vi "test6-AsteriskWildcardStatusRegistration.vi"(8 "error in (no error)":errorcluster, 11 "TestCase in":refnum<class "testcase-CSMBroadcast.lvclass">) -> (0 "error out":errorcluster, 3 "TestCase out":refnum<class "testcase-CSMBroadcast.lvclass">)   [LabVIEW 2017, in "testcase-CSMBroadcast.lvclass"]
uses:
  testcase-CSMBroadcast.lvclass
  0c20cacf-7d77-4f8e-aec5-f22e7d09936d.vi
  26de337d-8090-412f-9da5-e117a55d4726.vi
  de10340a-d592-45ad-b055-7fa7b377c551.vi
  e3eae2f8-d8ce-4adb-8167-9a417250fce1.vi
  a4d00e00-a9ed-4631-bf53-269bf71f16fc.vi
  src/user.lib/_NEVSTOP/Communicable State Machine(CSM)/AdvanceAPI/CSM - Revert Arguments-Safe String.vi
  src/user.lib/_NEVSTOP/Communicable State Machine(CSM)/AdvanceAPI/CSM - Make String Arguments Safe.vi
  src/user.lib/_NEVSTOP/Communicable State Machine(CSM)/AdvanceAPI/CSM - Break Down Multiple States String.vi
  src/user.lib/_NEVSTOP/Communicable State Machine(CSM)/AdvanceAPI/CSM - Compact Multiple States.vi
  src/user.lib/_NEVSTOP/Communicable State Machine(CSM)/AdvanceAPI/CSM - Keywords.vi
  src/user.lib/_NEVSTOP/Communicable State Machine(CSM)/_Shared/Trim Single-line Text.vi
  src/user.lib/_NEVSTOP/Communicable State Machine(CSM)/AdvanceAPI/CSM - Set Module Attribute.vi
  src/user.lib/_NEVSTOP/Communicable State Machine(CSM)/AdvanceAPI/CSM - Get Module Attribute.vi
  <vilib>/addons/_JKI Toolkits/VI Tester/TestCase.llb/TestCase.lvclass
  src/user.lib/_NEVSTOP/Communicable State Machine(CSM)/Communicable State Machine.lvlib
  CSM/CSM-Testcase.lvlib
  C:/Program Files (x86)/National Instruments/LabVIEW 2017/vi.lib/addons/_JKI Toolkits/VI Tester/TestCase.llb/TestCase.lvclass
panel:
  out "Execution Times":i32
  out "State History":string
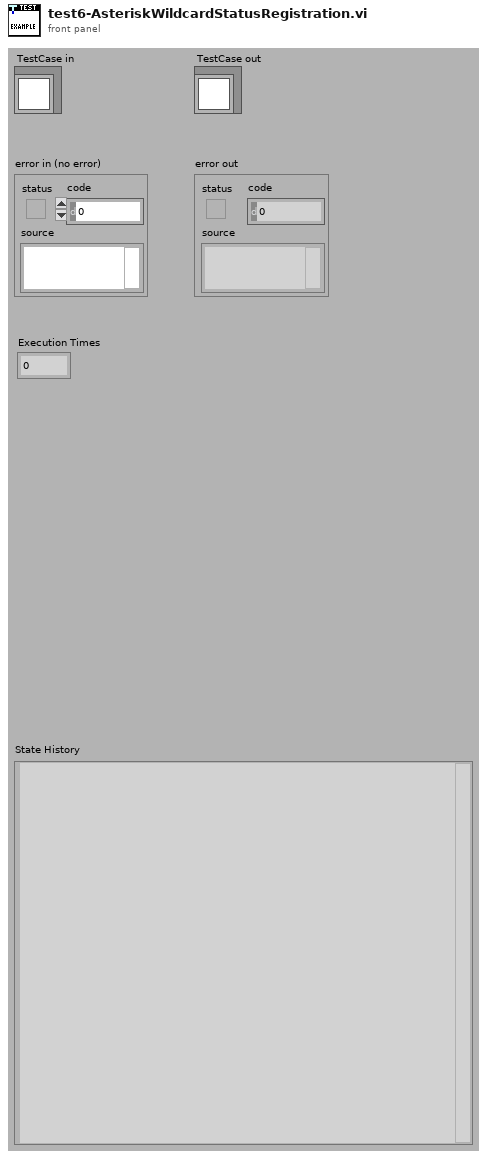
[diagram p1: front panel]
types:
  T1 = enum32{"Invalid", "Standard", "Closed", "Hidden", "Minimized", "Maximized"}
  T2 = enum32{"invalid app kind", "Development System", "Run Time System", "Student Edition", "Embedded LabVIEW", "Evaluation", "Custom"}
  T3 = typedef "Communicable State Machine.lvlib/_CSM_Response Source Message.ctl" = cluster{"‘State":string, "’Arguments":string, "’Error":errorcluster}
  T4 = cluster{"Current VI Reference":refnum<vi>, "Close Panel on Exit?":bool}
  T5 = cluster{"Core":cluster{"Current VI Reference":refnum<vi>, "Close Panel on Exit?":bool}, "Your Boolean data":bool, "Your string data":string, "TestData":i32}
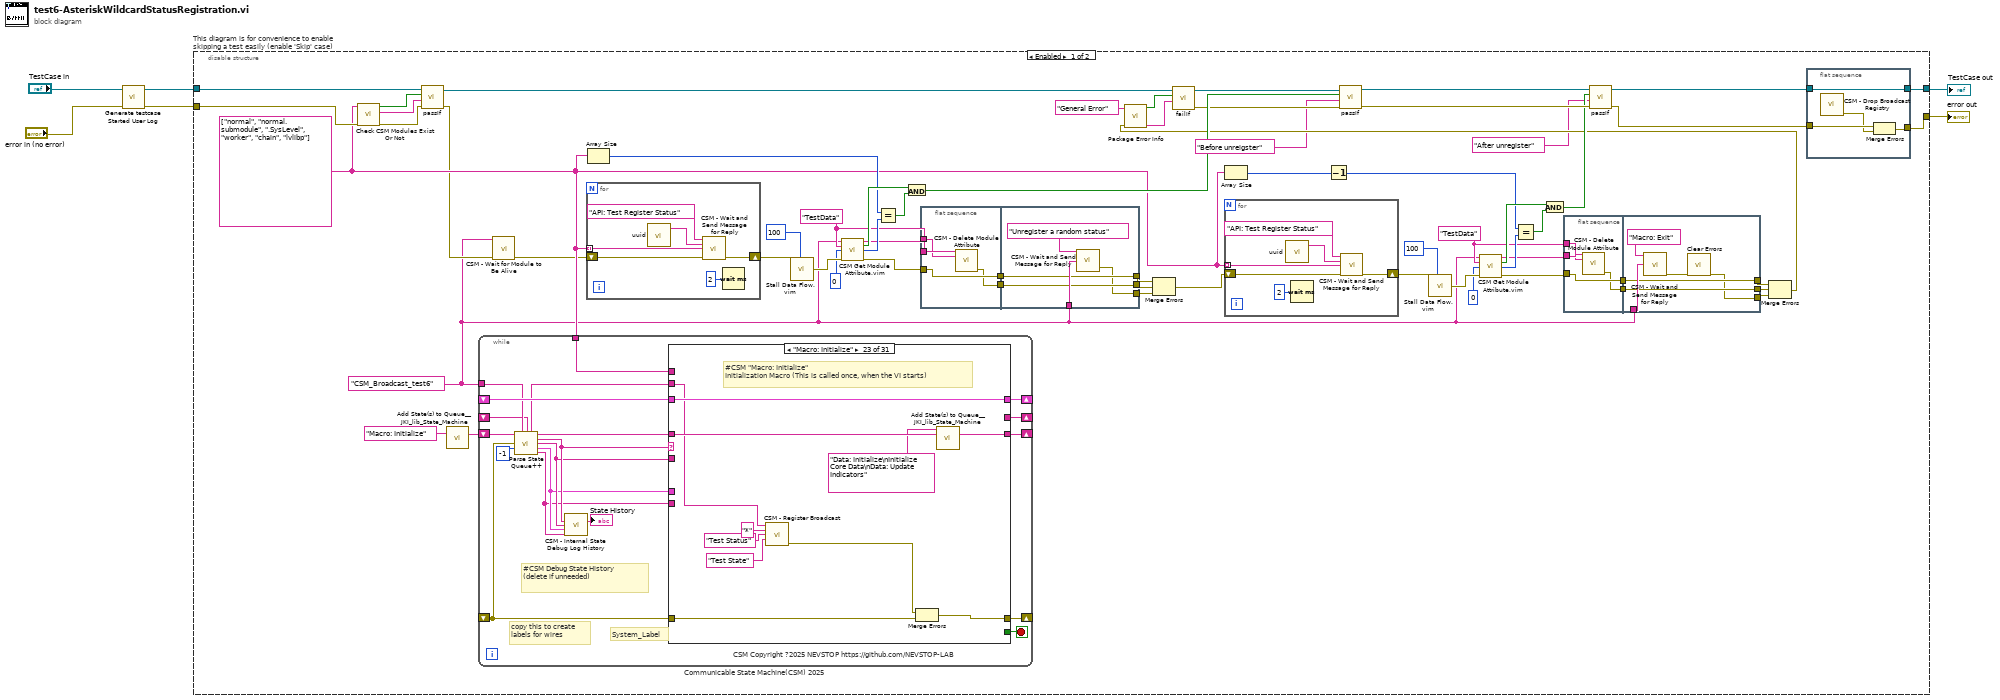
[diagram p0: block diagram]
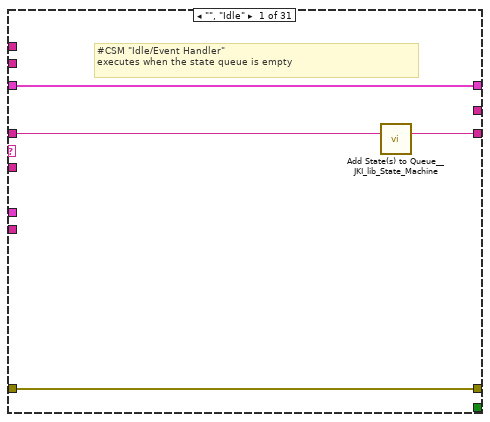
[diagram p2: hidden frame]
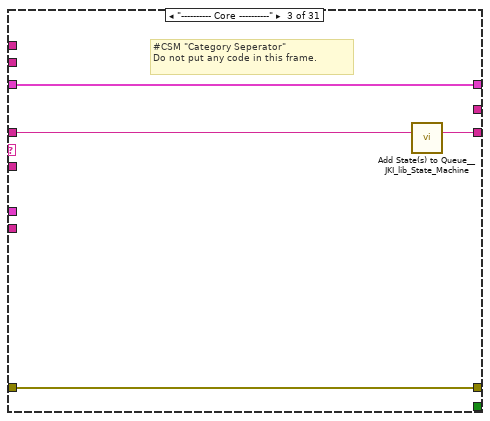
[diagram p4: hidden frame]
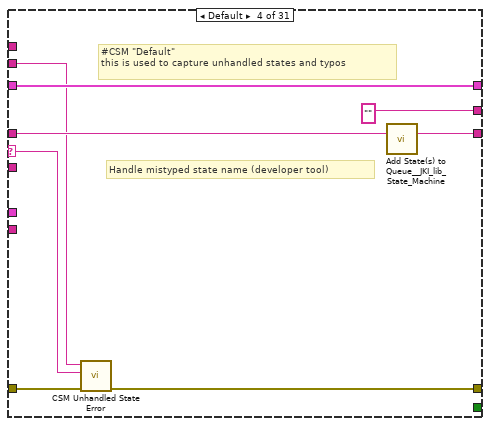
[diagram p5: hidden frame]
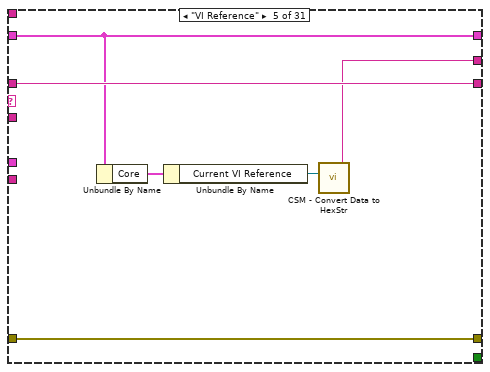
[diagram p6: hidden frame]
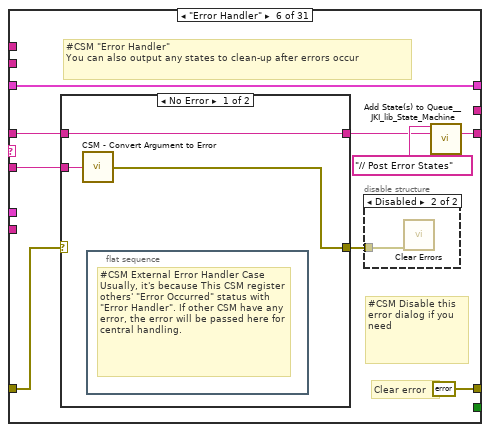
[diagram p7: hidden frame]
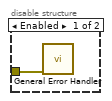
[diagram p8: hidden frame]
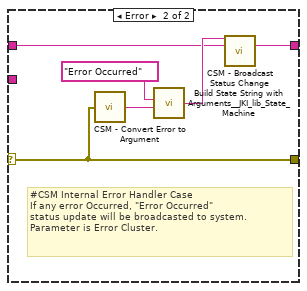
[diagram p9: hidden frame]
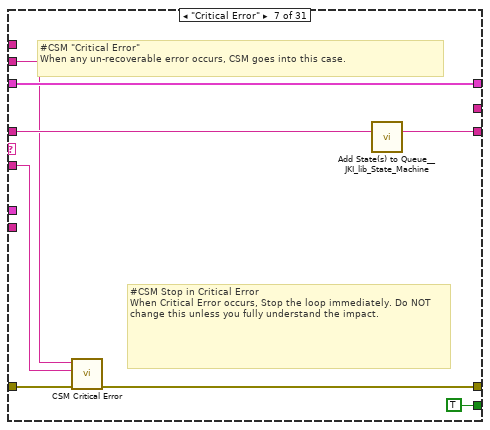
[diagram p10: hidden frame]
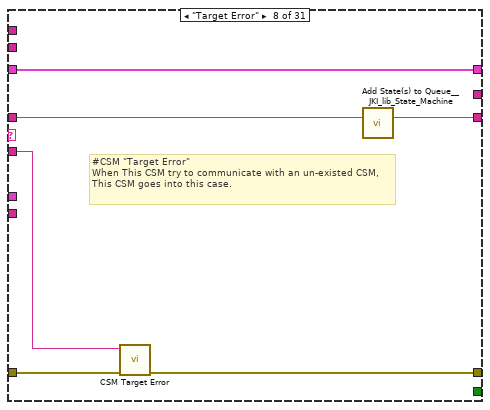
[diagram p11: hidden frame]
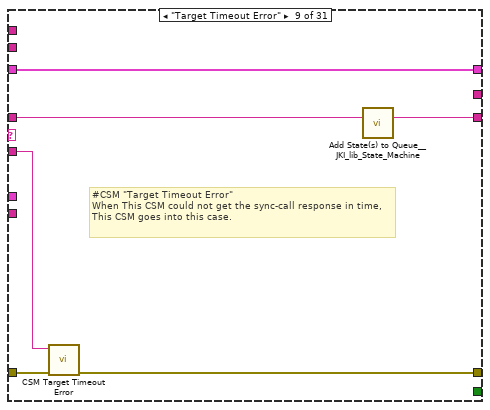
[diagram p12: hidden frame]
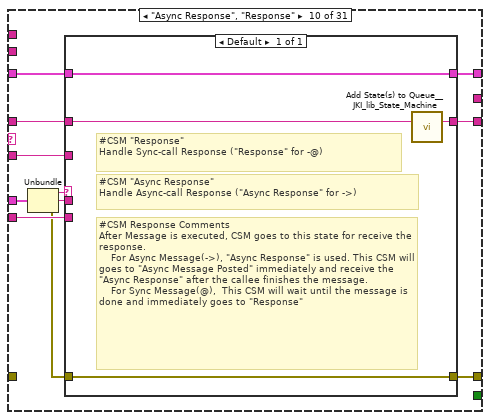
[diagram p13: hidden frame]
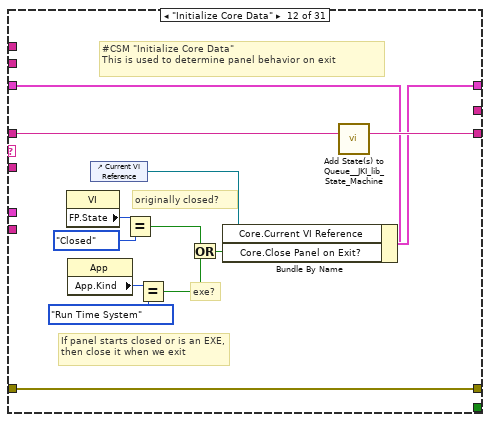
[diagram p15: hidden frame]
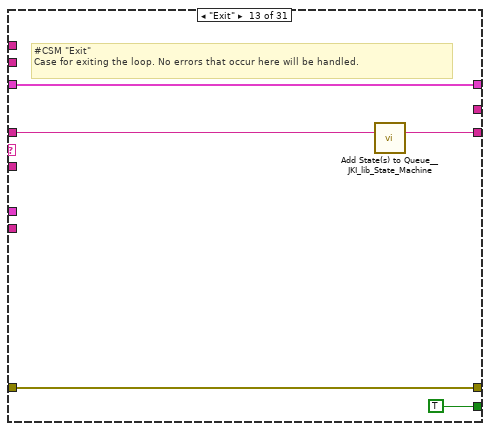
[diagram p16: hidden frame]
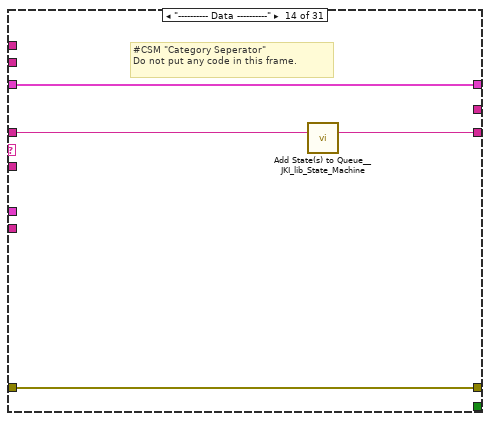
[diagram p17: hidden frame]
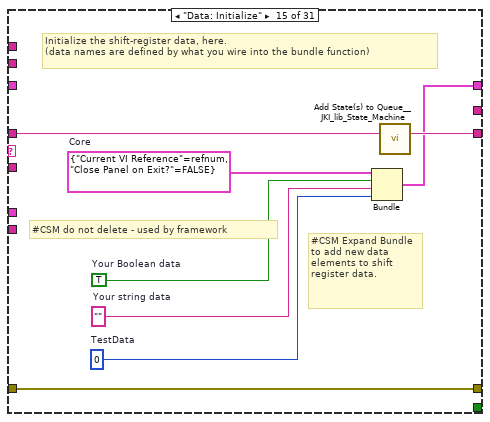
[diagram p18: hidden frame]
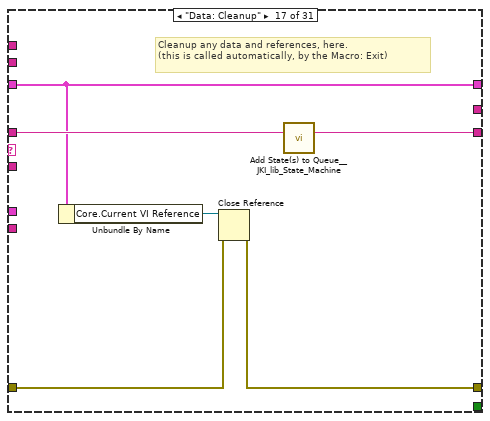
[diagram p20: hidden frame]
diagram:
  n1 = call "Generate testcase Started User Log.vi"("Error In"="error in (no error)") -> ("error out"=w1:errorcluster)  [unwired: 10 in]
  n2 = disable-structure "This diagram is for convenience to enable skipping a test easily (enable 'Skip' case)" shown="Enabled" {
    disable-tunnel: "TestCase in" -> [w24 w422]
    disable-tunnel: [w19 w420] -> w2
    disable-tunnel: [w18 w421] -> w4
    disable-tunnel: w1 -> [w23 w419]
    frame Enabled {
      w33 = "TestData" ("Attribute")
      w55 = "TestData" ("Attribute")
      w6 = "CSM_Broadcast_test6" ("Name (\"\" to Use UUID)")
      w22 = string[] ["normal", "normal.submodule", ".SysLevel", "worker", "chain", "lvlibp"]
      n3 = call "Check CSM Modules Exist Or Not.vi"("error in"=w23, "CSM names in"=w22) -> ("error out"=w25:errorcluster, "Debug string"=w26:string, "All Modules Exist?"=w27:bool)  [unwired: 7 in]
      n4 = call-dynamic "passIf.vi"("error in (no error)"=w25, "message (\"\")"=w26, "pass"=w27, "TestCase in"=w24) -> ("error out"=w8:errorcluster, "TestCase out"=w16:refnum<class "testcase-CSMBroadcast.lvclass">)  [unwired: 6 in]
      n5 = call <vilib>:"Add State(s) to Queue__JKI_lib_State_Machine.vi"("State(s) in (\"\")"="Macro: Initialize" ("Init State(\"Macro: Initialize\")")) -> ("States Out"=w66:string)  [unwired: 14 in]
      n6 = while "Communicable State Machine(CSM) 2025" {
        shift-right: [w110] -> _
        shift-left: _ -> [w109]
        shift-right: [w113] -> _
        shift-left: _ -> [w108]
        shift-right: [w112] -> _
        shift-left: w66 -> [w114]
        tunnel: w6 -> [w106]
        shift-right: [w107] -> _
        shift-left: _ -> [w100]
        tunnel: w22 -> [w97]
        stop <- w111 stop-if-true
        # "#CSM Debug State History\n(delete if unneeded)"
        # "copy this to create labels for wires"
        # "System_Label"
        # "CSM Copyright ?2025 NEVSTOP https://github.com/NEVSTOP-LAB"
        n7 = call "Parse State Queue++.vi"("State Queue"=w114, "Name (\"\" to Use UUID)"=w106, "Response Arguments"=w100, "Previous Error"=w108, "Dequeue (1 ms)"=-1 ("Timeout")) -> ("Name Used"=w101:string, "Remaining States"=w115:string, "Current State"=w105:string, "Arguments"=w104:string, "Additional Information"=w103:T3, "Source CSM"=w102:string)  [unwired: 5 in]
        n8 = call "CSM - Internal State Debug Log History.vi"("State"=w105, "Arguments (\"\")"=w104, ">> Response Source Message >>"=w103, "Source (\"\")"=w102) -> ("Debug Log"=→"State History":string)  [unwired: 11 in]
        n9 = case shown="\"Macro: Initialize\"" w105 {
          selector: w105 -> [_ _ _ w129 _ _ _ _ _ _ _ _ _ _ _ _ _ _ _ _ _ _ _ _ _ _ _ _ _ _ _]
          tunnel: w115 -> [w116 w121 w126 w133 w139 w145 w166 w172 w178 w186 w197 w211 w216 w220 w228 w230 w237 w241 w245 w251 w266 w335 w346 w359 w361 w365 w370 w377 w381 w392 w412]
          tunnel: w104 -> [_ _ _ _ _ w144 w162 w171 w176 w185 _ _ _ _ _ _ _ _ _ w246 w260 _ _ _ _ _ w368 _ _ _ _]
          tunnel: w109 -> [w117 w120 w123 w131 w138 w148 w167 w173 w179 w188 w196 w204 w214 w217 _ w229 w232 w238 w243 w249 w262 w332 w343 w356 w360 w364 w369 w374 w378 w384 w398]
          tunnel: [w118 w122 w124 w127 w140 errorcluster {"status"=FALSE, "code"=0, "source"=""} ("error out") w163 w169 w175 w191 w198 w208 w213 w218 w225 w231 w233 w239 w242 w247 w263 w333 w337 w348 w362 w366 w371 w375 w379 w386 w400] -> w113
          tunnel: w108 -> [w118 w122 w124 w134 w140 w146 w168 w170 w177 _ w198 w208 w213 w218 w225 w231 w234 w239 w242 w248 w264 w333 w344 w357 w362 w366 w371 w375 w379 w390 w410]
          tunnel: [w119 w121 w125 w132 w139 w141 w165 w174 w180 w187 w197 w210 w215 w219 w227 w230 w236 w240 w244 w250 w265 w334 w345 w358 w361 w365 w370 w376 w380 w391 w411] -> w112
          tunnel: [_ _ _ _ _ _ TRUE _ _ _ _ _ TRUE _ _ _ _ _ _ _ _ _ _ _ _ _ _ _ _ _ _] -> w111
          tunnel: [w117 w120 w123 w131 w138 w148 w167 w173 w179 w189 w196 w209 w214 w217 w226 w229 w232 w238 w243 w249 w262 w332 w343 w356 w360 w364 w369 w374 w378 w388 w396] -> w110
          tunnel: w102 -> [_ _ _ _ _ _ _ _ _ w183 _ _ _ _ _ _ _ _ _ _ _ _ _ _ _ _ _ _ _ _ _]
          tunnel: w103 -> [_ _ _ _ _ _ _ _ _ w190 _ _ _ _ _ _ _ _ _ _ _ _ _ _ _ _ _ _ _ _ _]
          tunnel: [_ _ _ "" w135 _ _ _ _ _ _ _ _ _ _ _ _ _ _ _ _ _ _ _ _ "API1 Response" w367 _ _ _ _] -> w107
          tunnel: w101 -> [_ _ _ w128 _ _ w161 _ _ _ _ _ _ _ _ _ _ _ _ _ _ _ w338 w350 _ _ _ _ _ w387 w407]
          tunnel: w97 -> [_ _ _ _ _ _ _ _ _ _ _ _ _ _ _ _ _ _ _ _ _ _ _ _ _ _ _ _ _ _ w403]
          frame "", "Idle" {
            # "#CSM \"Idle/Event Handler\"\nexecutes when the state queue is empty"
            n10 = call <vilib>:"Add State(s) to Queue__JKI_lib_State_Machine.vi"("State(s) in (\"\")"=w116) -> ("States Out"=w119:string)  [unwired: 14 in]
          }
          frame "CSM Documentation" {
            # "#CSM README FIRST\n\nCommunicable State Machine(CSM) is a LabVIEW application framework that builds upon JKI State Machine(JKISM). It follows the pattern of JKISM and extends the keywords to describe message communication between modules, including concepts such as Sync-Message, Async-Message, Subscription/Unsubscription of status - essential elements for creating reusable code modules. For more information, please visit the CSM wiki: https://nevstop-lab.github.io/CSM-Wiki/\n\nFor instructions on JKI State Machine, visit: http://jki.net/state-machine/\nFor information about CSM, visit: https://github.com/NEVSTOP-LAB"
            # "#CSM \"Documentation\"\nCase for holding CSM Documenation"
          }
          frame "---------- Core ----------" {
            # "#CSM \"Category Seperator\"\nDo not put any code in this frame."
            n11 = call <vilib>:"Add State(s) to Queue__JKI_lib_State_Machine.vi"("State(s) in (\"\")"=w126) -> ("States Out"=w125:string)  [unwired: 14 in]
          }
          frame Default {
            # "#CSM \"Default\"\nthis is used to capture unhandled states and typos"
            # "Handle mistyped state name (developer tool)"
            n12 = call "CSM Unhandled State Error.vi"("error in (no error)"=w134, "Undefined State"=w129, "CSM Name"=w128) -> ("error out"=w127:errorcluster)  [unwired: 8 in]
            n13 = call <vilib>:"Add State(s) to Queue__JKI_lib_State_Machine.vi"("State(s) in (\"\")"=w133) -> ("States Out"=w132:string)  [unwired: 14 in]
          }
          frame "VI Reference" {
            n14 = Unbundle By Name(w138) -> ("Core"=w137:T4)
            n15 = Unbundle By Name(w137) -> ("Current VI Reference"=w136:refnum<vi>)
            n16 = call "CSM - Convert Data to HexStr.vi"("Variant"=w136) -> ("HEX String (0-9,A-F)"=w135:string)  [unwired: 8 in]
          }
          frame "Error Handler" {
            # "#CSM Disable this error dialog if you need"
            # "#CSM \"Error Handler\"\nYou can also output any states to clean-up after errors occur"
            # "Clear error"
            n17 = case shown="No Error" w146 {
              selector: w146 -> [_ w155]
              tunnel: [w154 w157] -> w142
              tunnel: w145 -> [w154 w156]
              tunnel: w144 -> [w153 _]
              tunnel: [w152 w155] -> w147
              frame No Error {
                n18 = call "CSM - Convert Argument to Error.vi"("Argument"=w153) -> ("Error"=w152:errorcluster)  [unwired: 4 in]
                n19 = flat-sequence {
                  frame #0 {
                    # "#CSM External Error Handler Case\nUsually, it's because This CSM register others' \"Error Occurred\" status with \"Error Handler\". If other CSM have any error, the error will be passed here for central handling."
                  }
                }
              }
              frame Error {
                # "#CSM Internal Error Handler Case \nIf any error Occurred, \"Error Occurred\" \nstatus update will be broadcasted to system.\nParameter is Error Cluster."
                n20 = call "CSM - Convert Error to Argument.vi"("Error"=w155) -> ("Argument"=w159:string)  [unwired: 4 in]
                n21 = call <vilib>:"Build State String with Arguments__JKI_lib_State_Machine.vi"("Arguments (\"\")"=w159, "State"="Error Occurred" ("Status with Arguments")) -> ("State with Arguments"=w158:string)  [unwired: 4 in]
                n22 = call "CSM - Broadcast Status Change.vi"("Status With Arguments"=w158, "State Queue"=w156) -> ("Remaining States"=w157:string)  [unwired: 13 in]
              }
            }
            n23 = disable-structure shown="Disabled" {
              disable-tunnel: w147 -> [w150 w151]
              frame Enabled {
                n24 = call <vilib>:"General Error Handler.vi"("error in (no error)"=w150) -> ()  [unwired: 10 in, 5 out]
              }
              frame Disabled {
                n25 = call <vilib>:"Clear Errors.vi"("error in (no error)"=w151) -> ()  [unwired: 5 in, 2 out]
              }
            }
            n26 = call <vilib>:"Add State(s) to Queue__JKI_lib_State_Machine.vi"("State(s) in Front (\"\")"="// Post Error States", "State(s) in (\"\")"=w142) -> ("States Out"=w141:string)  [unwired: 13 in]
          }
          frame "Critical Error" {
            # "#CSM Stop in Critical Error\nWhen Critical Error occurs, Stop the loop immediately. Do NOT change this unless you fully understand the impact."
            # "#CSM \"Critical Error\"\nWhen any un-recoverable error occurs, CSM goes into this case."
            n27 = call "CSM Critical Error.vi"("error in (no error)"=w168, "Arugments (As Reason)"=w162, "CSM Name"=w161) -> ("error out"=w163:errorcluster)  [unwired: 8 in]
            n28 = call <vilib>:"Add State(s) to Queue__JKI_lib_State_Machine.vi"("State(s) in (\"\")"=w166) -> ("States Out"=w165:string)  [unwired: 14 in]
          }
          frame "Target Error" {
            # "#CSM \"Target Error\"\nWhen This CSM try to communicate with an un-existed CSM, This CSM goes into this case."
            n29 = call "CSM Target Error.vi"("error in (no error)"=w170, "Arguments (As CSM Name)"=w171) -> ("error out"=w169:errorcluster)  [unwired: 9 in]
            n30 = call <vilib>:"Add State(s) to Queue__JKI_lib_State_Machine.vi"("State(s) in (\"\")"=w172) -> ("States Out"=w174:string)  [unwired: 14 in]
          }
          frame "Target Timeout Error" {
            # "#CSM \"Target Timeout Error\"\nWhen This CSM could not get the sync-call response in time, This CSM goes into this case."
            n31 = call "CSM Target Timeout Error.vi"("error in (no error)"=w177, "Arguments (As CSM Name)"=w176) -> ("error out"=w175:errorcluster)  [unwired: 9 in]
            n32 = call <vilib>:"Add State(s) to Queue__JKI_lib_State_Machine.vi"("State(s) in (\"\")"=w178) -> ("States Out"=w180:string)  [unwired: 14 in]
          }
          frame "Async Response", "Response" {
            n33 = Unbundle(w190) -> ("‘State"=w184:string, "’Arguments"=w182:string, "’Error"=w181:errorcluster)
            n34 = case shown="Default" w184 {
              tunnel: [w195] -> w191
              tunnel: w181 -> [w195]
              tunnel: [w194] -> w189
              tunnel: w188 -> [w194]
              tunnel: [w192] -> w187
              tunnel: w186 -> [w193]
              tunnel: w185 -> [_]
              tunnel: w183 -> [_]
              tunnel: w182 -> [_]
              frame Default {
                # "#CSM Response Comments\nAfter Message is executed, CSM goes to this state for receive the response.\n    For Async Message(->), \"Async Response\" is used. This CSM will goes to \"Async Message Posted\" immediately and receive the \"Async Response\" after the callee finishes the message.\n    For Sync Message(@),  This CSM will wait until the message is done and immediately goes to \"Response\""
                # "#CSM \"Async Response\"\nHandle Async-call Response (\"Async Response\" for ->)"
                # "#CSM \"Response\"\nHandle Sync-call Response (\"Response\" for -@)"
                n35 = call <vilib>:"Add State(s) to Queue__JKI_lib_State_Machine.vi"("State(s) in (\"\")"=w193) -> ("States Out"=w192:string)  [unwired: 14 in]
              }
            }
          }
          frame "Async Message Posted" {
            # "#CSM \"Async Message Posted\"\nAfter Async Message is posted (-> or ->| ), CSM goes to this state for post-action.\nYou can use Argument - State to tell which Async Message is called."
          }
          frame "Initialize Core Data" {
            # "#CSM \"Initialize Core Data\"\nThis is used to determine panel behavior on exit"
            # "originally closed?"
            # "exe?"
            # "If panel starts closed or is an EXE, then close it when we exit"
            n36 = property class="VI"() -> ("FP.State"=w201:T1)  [unwired: 2 in, 2 out]
            n37 = property class="App"() -> ("App.Kind"=w207:T2)  [unwired: 2 in, 2 out]
            n38 = control-ref of="Current VI Reference"() -> (w202:refnum<vi>)
            n39 = Equal?(x=w201, y=T1."Closed" ("Front Panel Window:State")) -> (x = y?=w199:bool)
            n40 = Equal?(x=w207, y=T2."Run Time System" ("Application:Kind")) -> (x = y?=w205:bool)
            n41 = Or(x=w199, y=w205) -> (x .or. y?=w203:bool)
            n42 = Bundle By Name(cluster=w204, "Core.Current VI Reference"=w202, "Core.Close Panel on Exit?"=w203) -> (w209:T5)
            n43 = call <vilib>:"Add State(s) to Queue__JKI_lib_State_Machine.vi"("State(s) in (\"\")"=w211) -> ("States Out"=w210:string)  [unwired: 14 in]
          }
          frame "Exit" {
            # "#CSM \"Exit\"\nCase for exiting the loop. No errors that occur here will be handled."
            n44 = call <vilib>:"Add State(s) to Queue__JKI_lib_State_Machine.vi"("State(s) in (\"\")"=w216) -> ("States Out"=w215:string)  [unwired: 14 in]
          }
          frame "---------- Data ----------" {
            # "#CSM \"Category Seperator\"\nDo not put any code in this frame."
            n45 = call <vilib>:"Add State(s) to Queue__JKI_lib_State_Machine.vi"("State(s) in (\"\")"=w220) -> ("States Out"=w219:string)  [unwired: 14 in]
          }
          frame "Data: Initialize" {
            w221 = 0  # TestData
            w222 = T4 {"Current VI Reference"=refnum, "Close Panel on Exit?"=FALSE}  # Core
            w224 = TRUE  # Your Boolean data
            w223 = ""  # Your string data
            # "#CSM do not delete - used by framework"
            # "#CSM Expand Bundle to add new data elements to shift register data."
            # "Initialize the shift-register data, here.\n(data names are defined by what you wire into the bundle function)"
            n46 = Bundle("Core"=w222, "Your Boolean data"=w224, "Your string data"=w223, "TestData"=w221) -> (w226:T5)  [unwired: 1 in]
            n47 = call <vilib>:"Add State(s) to Queue__JKI_lib_State_Machine.vi"("State(s) in (\"\")"=w228) -> ("States Out"=w227:string)  [unwired: 14 in]
          }
          frame "Data: Update Indicators" {
          }
          frame "Data: Cleanup" {
            # "Cleanup any data and references, here.\n(this is called automatically, by the Macro: Exit)"
            n48 = Unbundle By Name(w232) -> ("Core.Current VI Reference"=w235:refnum<vi>)
            n49 = Close Reference(reference=w235, error in (no error)=w234) -> (error out=w233:errorcluster)
            n50 = call <vilib>:"Add State(s) to Queue__JKI_lib_State_Machine.vi"("State(s) in (\"\")"=w237) -> ("States Out"=w236:string)  [unwired: 14 in]
          }
          frame "---------- UI ----------" {
            # "#CSM \"Category Seperator\"\nDo not put any code in this frame."
            n51 = call <vilib>:"Add State(s) to Queue__JKI_lib_State_Machine.vi"("State(s) in (\"\")"=w241) -> ("States Out"=w240:string)  [unwired: 14 in]
          }
          frame "UI: Initialize" {
            # "#CSM \"UI: Initialize\"\nInitialize the User Interface, here.\n(this is called automatically, by the Macro: Init)"
            n52 = call <vilib>:"Add State(s) to Queue__JKI_lib_State_Machine.vi"("State(s) in (\"\")"=w245) -> ("States Out"=w244:string)  [unwired: 14 in]
          }
          frame "UI: Cursor Set" {
            # "#CSM \"UI: Cursor Set\"\nSet and Unset Cursor Busy.\n(Usage: \"UI: Cursor Set >> Busy|Idle\")"
            # "Argument"
            n53 = disable-structure shown="TARGET_TYPE!=Windows" {
              disable-tunnel: w248 -> [w254 w259]
              disable-tunnel: [w253 w259] -> w247
              disable-tunnel: w246 -> [w252 _]
              frame condition #0 (active) {
                n54 = case shown="\"Idle\", Default" w252 {
                  tunnel: w254 -> [w256 w258]
                  tunnel: [w255 w257] -> w253
                  frame "Idle", Default {
                    n55 = call <vilib>:"Unset Busy.vi"("error in (no error)"=w256) -> ("error out"=w255:errorcluster)  [unwired: 10 in]
                  }
                  frame "Busy" {
                    n56 = call <vilib>:"Set Busy.vi"("error in (no error)"=w258) -> ("error out"=w257:errorcluster)  [unwired: 9 in, 1 out]
                  }
                }
              }
              frame condition #1 {
              }
            }
            n57 = call <vilib>:"Add State(s) to Queue__JKI_lib_State_Machine.vi"("State(s) in (\"\")"=w251) -> ("States Out"=w250:string)  [unwired: 14 in]
          }
          frame "UI: Front Panel State" {
            # "#CSM \"UI: Front Panel State\"\nSet Front Panel Open or Closed\n(Usage: \"UI: Front Panel State >> Open|Close\")"
            # "Argument"
            n58 = Unbundle By Name(w262) -> ("Core.Current VI Reference"=w261:refnum<vi>)
            n59 = call <vilib>:"Add State(s) to Queue__JKI_lib_State_Machine.vi"("State(s) in (\"\")"=w266) -> ("States Out"=w265:string)  [unwired: 14 in]
            n60 = case shown="\"Close\", \"Closed\"" w260 {
              tunnel: w264 -> [w272 w287 w298 w311 w324]
              tunnel: [w274 w288 w300 w313 w326] -> w263
              tunnel: w261 -> [w273 w285 w299 w312 w325]
              frame "Open", "Standard", Default {
                w267 = T1."Standard" ("State")
                n61 = property class="VI"(reference=w273, error in=w272) -> (reference out=w270:refnum<vi>, error out=w271:errorcluster, "FP.State"=w269:T1)
                n62 = Not Equal?(x=w269, y=w267) -> (x != y?=w268:bool)
                n63 = case shown="True" w268 {
                  tunnel: [w278 w280] -> w274
                  tunnel: w271 -> [w277 w280]
                  tunnel: w270 -> [w276 _]
                  tunnel: w267 -> [w275 _]
                  frame True {
                    n64 = invoke class="VI" method="FP.Open"(reference=w276, error in=w277, "Activate"=TRUE, "State"=w275) -> (error out=w278:errorcluster)  [unwired: 1 in, 4 out]
                  }
                  frame False {
                  }
                }
              }
              frame "Close", "Closed" {
                n65 = property class="VI"(reference=w285, error in=w287) -> (reference out=w284:refnum<vi>, error out=w286:errorcluster, "FP.State"=w282:T1)
                n66 = Not Equal?(x=w282, y=T1."Closed" ("Front Panel Window:State")) -> (x != y?=w281:bool)
                n67 = case shown="False" w281 {
                  tunnel: [w289 w292] -> w288
                  tunnel: w286 -> [w289 w291]
                  tunnel: w284 -> [_ w290]
                  frame False {
                  }
                  frame True {
                    n68 = invoke class="VI" method="FP.Close"(reference=w290, error in=w291) -> (error out=w292:errorcluster)  [unwired: 1 in, 2 out]
                  }
                }
              }
              frame "Hidden", "Hide" {
                w293 = T1."Hidden" ("State")
                n69 = property class="VI"(reference=w299, error in=w298) -> (reference out=w296:refnum<vi>, error out=w297:errorcluster, "FP.State"=w295:T1)
                n70 = Not Equal?(x=w295, y=w293) -> (x != y?=w294:bool)
                n71 = case shown="True" w294 {
                  tunnel: [w304 w305] -> w300
                  tunnel: w297 -> [w303 w305]
                  tunnel: w296 -> [w302 _]
                  tunnel: w293 -> [w301 _]
                  frame True {
                    n72 = invoke class="VI" method="FP.Open"(reference=w302, error in=w303, "State"=w301) -> (error out=w304:errorcluster)  [unwired: 2 in, 4 out]
                  }
                  frame False {
                  }
                }
              }
              frame "Minimize", "Minimized" {
                w306 = T1."Minimized" ("State")
                n73 = property class="VI"(reference=w312, error in=w311) -> (reference out=w309:refnum<vi>, error out=w310:errorcluster, "FP.State"=w308:T1)
                n74 = Not Equal?(x=w308, y=w306) -> (x != y?=w307:bool)
                n75 = case shown="True" w307 {
                  tunnel: [w317 w318] -> w313
                  tunnel: w310 -> [w316 w318]
                  tunnel: w309 -> [w315 _]
                  tunnel: w306 -> [w314 _]
                  frame True {
                    n76 = invoke class="VI" method="FP.Open"(reference=w315, error in=w316, "State"=w314) -> (error out=w317:errorcluster)  [unwired: 2 in, 4 out]
                  }
                  frame False {
                  }
                }
              }
              frame "Maximize", "Maximized" {
                w319 = T1."Maximized" ("State")
                n77 = property class="VI"(reference=w325, error in=w324) -> (reference out=w322:refnum<vi>, error out=w323:errorcluster, "FP.State"=w321:T1)
                n78 = Not Equal?(x=w321, y=w319) -> (x != y?=w320:bool)
                n79 = case shown="True" w320 {
                  tunnel: [w330 w331] -> w326
                  tunnel: w323 -> [w329 w331]
                  tunnel: w322 -> [w328 _]
                  tunnel: w319 -> [w327 _]
                  frame True {
                    n80 = invoke class="VI" method="FP.Open"(reference=w328, error in=w329, "State"=w327) -> (error out=w330:errorcluster)  [unwired: 2 in, 4 out]
                  }
                  frame False {
                  }
                }
              }
            }
          }
          frame "---------- Macro ----------" {
            # "#CSM \"Category Seperator\"\nDo not put any code in this frame."
            n81 = call <vilib>:"Add State(s) to Queue__JKI_lib_State_Machine.vi"("State(s) in (\"\")"=w335) -> ("States Out"=w334:string)  [unwired: 14 in]
          }
          frame "Macro: Initialize" {
            # "#CSM \"Macro: Initialize\"\nInitialization Macro (This is called once, when the VI starts)"
            n82 = call "CSM - Register Broadcast.vi"("CSM Name(Empty for Broadcast Event)"=w338, "Source CSM Name (* as Default)"="*", "Trigger"="Test Status" ("Status"), "API (If \"\", Same as Trigger)"="Test State" ("Response Message (If \"\", Same as Source Message)")) -> ("error out"=w336:errorcluster)  [unwired: 10 in, 1 out]
            n83 = Merge Errors(w336, w344) -> (w337:errorcluster)
            n84 = call <vilib>:"Add State(s) to Queue__JKI_lib_State_Machine.vi"("State(s) in Front (\"\")"="Data: Initialize\nInitialize Core Data\nData: Update Indicators", "State(s) in (\"\")"=w346) -> ("States Out"=w345:string)  [unwired: 13 in]
          }
          frame "Macro: Exit" {
            # "#CSM \"Macro: Exit\"\nExit Macro (This is called once, when the VI exits)"
            n85 = call "CSM - Unregister Broadcast.vi"("CSM Name(Empty for Broadcast Event)"=w350, "Source CSM Name (* as Default)"="*", "Trigger"="Test Status" ("Status"), "API (\"*\" as Default)"="Test State" ("Response Message (If \"\", Same as Source Message)")) -> ("error out"=w347:errorcluster)  [unwired: 10 in, 1 out]
            n86 = call <vilib>:"Add State(s) to Queue__JKI_lib_State_Machine.vi"("State(s) in Front (\"\")"="//Exit Sub-Modules ", "State(s) at Back (\"\")"="Data: Cleanup\nExit") -> ("States Out"=w354:string)  [unwired: 13 in]
            n87 = Merge Errors(w347, w357) -> (w348:errorcluster)
            n88 = call <vilib>:"Add State(s) to Queue__JKI_lib_State_Machine.vi"("State(s) in Front (\"\")"=w354, "State(s) in (\"\")"=w359) -> ("States Out"=w358:string)  [unwired: 13 in]
          }
          frame "---------- API ----------" {
            # "#CSM \"Category Seperator\"\nDo not put any code in this frame."
          }
          frame "API: API1" {
            # "#CSM API Example\nCopy/Rename this case for your own API"
            # "#CSM Response\nConnect this to return the response of your API"
            # "#CSM >> Msg/Rep's CSM >>\nIf you need to tell who triggered this state , use this string. If it's this case itself, this string is \"\"."
            # "#CSM >> Arguments >>\nDeal with the parameter if any"
          }
          frame "API: API2" {
            # "#CSM API Example\nCopy/Rename this case for your own API"
            # "unpack Hex String  to Variant\nif complex parameter is needed."
            n89 = call "CSM - Convert HexStr to Data.vi"("HEX String"=w368) -> ()  [unwired: 7 in, 2 out]
            n90 = disable-structure shown="Disabled" {
              disable-tunnel: [w372 "API2 Response"] -> w367
              frame Disabled {
                # "pack variant to hexstr \nif complex response is needed."
                # "complex Response"
                n91 = call "CSM - Convert Data to HexStr.vi"() -> ("HEX String (0-9,A-F)"=w372:string)  [unwired: 9 in]
              }
              frame Enabled {
              }
            }
          }
          frame "---------- Action ----------" {
            # "#CSM \"Category Seperator\"\nDo not put any code in this frame."
            n92 = call <vilib>:"Add State(s) to Queue__JKI_lib_State_Machine.vi"("State(s) in (\"\")"=w377) -> ("States Out"=w376:string)  [unwired: 14 in]
          }
          frame "Action: action1" {
            # "#CSM \"Internal State\"\nThis category is used for holding internal states"
            n93 = call <vilib>:"Add State(s) to Queue__JKI_lib_State_Machine.vi"("State(s) in (\"\")"=w381) -> ("States Out"=w380:string)  [unwired: 14 in]
          }
          frame "Test State" {
            n94 = Unbundle By Name(w384) -> ("TestData"=w389:i32)
            n95 = disable-structure shown="Enabled" {
              frame Disabled {
                n96 = feedback #1(0 ("y")) -> (w394:i32)
                n97 = Increment(x=w394) -> (x+1=w393:i32)
                "Execution Times" <- w393
                n98 = feedback-in #1(w393) -> ()
              }
              frame Enabled {
              }
            }
            n99 = Increment(x=w389) -> (x+1=w382:i32)
            n100 = Bundle By Name(cluster=w384, "TestData"=w382) -> (w388:T5)
            n101 = call "CSM Set Module Attribute.vim"("CSM Name"=w387, "Attribute"="TestData", "Value"=w382) -> ("error out"=w385:errorcluster)  [unwired: 9 in, 3 out]
            n102 = call <vilib>:"Add State(s) to Queue__JKI_lib_State_Machine.vi"("State(s) in (\"\")"=w392) -> ("States Out"=w391:string)  [unwired: 14 in]
            n103 = Merge Errors(w390, w385) -> (w386:errorcluster)
          }
          frame "Unregister a random status" {
            n104 = Random Number (0-1)() -> (number: 0 to 1=w405:dbl)
            n105 = Array Size(array=w403) -> (size(s)=w406:i32)
            n106 = Multiply(x=w406, y=w405) -> (x*y=w404:dbl)
            n107 = Bundle By Name(cluster=w398, "TestData"=0) -> (w396:T5)
            n108 = Round Toward -Infinity(1:w404) -> (0:w402:dbl)
            n109 = Index Array(array=w403, index=w402) -> (element=w401:string)
            n110 = call "CSM - Unregister Broadcast.vi"("CSM Name(Empty for Broadcast Event)"=w407, "Source CSM Name (* as Default)"=w401, "Trigger"="Test Status" ("Status"), "API (\"*\" as Default)"="Test State" ("Response Message (If \"\", Same as Source Message)")) -> ("error out"=w399:errorcluster)  [unwired: 10 in, 1 out]
            n111 = Merge Errors(w410, w399) -> (w400:errorcluster)
            n112 = call <vilib>:"Add State(s) to Queue__JKI_lib_State_Machine.vi"("State(s) in (\"\")"=w412) -> ("States Out"=w411:string)  [unwired: 14 in]
          }
        }
      }
      n113 = call "CSM - Wait for Module to Be Alive.vi"("CSM Name"=w6, "error in (no error)"=w8) -> ("error out"=w7:errorcluster)  [unwired: 11 in, 2 out]
      n114 = for {
        tunnel: w22 -> [w416] mode=indexing
        shift-right: [w415] -> w64
        shift-left: w7 -> [w414]
        n115 = call "uuid.vi"() -> ("UUID"=w417:string)  [unwired: 11 in]
        n116 = call "CSM - Wait and Send Message for Reply.vi"("State"="API: Test Register Status", "Arguments (\"\")"=w417, "Target Module"=w416, "Error In (No Error)"=w414) -> ("error out"=w415:errorcluster)  [unwired: 8 in, 3 out]
        n117 = Wait (ms)(milliseconds to wait=u32 2) -> ()  [unwired: 1 out]
      }
      n118 = Array Size(array=w22) -> (size(s)=w59:i32)
      n119 = call "Stall Data Flow.vim"("value in"=w64, "milliseconds to wait"=u32 100) -> ("value out"=w63:errorcluster)  [unwired: 1 out]
      n120 = call "CSM Get Module Attribute.vim"("CSM Name"=w6, "Attribute"=w55, "Default Value (Empty Variant)"=0 ("x+1"), "Error In"=w63) -> ("CSM Name (Dup)"=w56:string, "Found"=w61:bool, "Value"=w60:i32, "error out"=w54:errorcluster)  [unwired: 7 in, 1 out]
      n121 = Equal?(x=w59, y=w60) -> (x = y?=w58:bool)
      n122 = And(x=w61, y=w58) -> (x .and. y?=w57:bool)
      n123 = flat-sequence {
        tunnel: w56 -> [w91]
        tunnel: w55 -> [w90]
        tunnel: w54 -> [w89]
        tunnel: [w89] -> w53
        tunnel: [w88] -> w52
        tunnel: w6 -> [w95]
        tunnel: w53 -> [w94]
        tunnel: w52 -> [w93]
        tunnel: [w94] -> w51
        tunnel: [w93] -> w50
        tunnel: [w92] -> w49
        frame #0 {
          n124 = call "CSM - Delete Module Attribute.vi"("CSM Name"=w91, "Attribute"=w90) -> ("error out"=w88:errorcluster)  [unwired: 10 in, 3 out]
        }
        frame #1 {
          n125 = call "CSM - Wait and Send Message for Reply.vi"("State"="Unregister a random status", "Target Module"=w95) -> ("error out"=w92:errorcluster)  [unwired: 10 in, 3 out]
        }
      }
      n126 = Merge Errors(w51, w50, w49) -> (w41:errorcluster)
      n127 = for {
        tunnel: w22 -> [w85] mode=indexing
        shift-right: [w84] -> w47
        shift-left: w41 -> [w83]
        n128 = call "uuid.vi"() -> ("UUID"=w86:string)  [unwired: 11 in]
        n129 = Wait (ms)(milliseconds to wait=u32 2) -> ()  [unwired: 1 out]
        n130 = call "CSM - Wait and Send Message for Reply.vi"("State"="API: Test Register Status", "Arguments (\"\")"=w86, "Target Module"=w85, "Error In (No Error)"=w83) -> ("error out"=w84:errorcluster)  [unwired: 8 in, 3 out]
      }
      n131 = Array Size(array=w22) -> (size(s)=w40:i32)
      n132 = Decrement(x=w40) -> (x-1=w39:i32)
      n133 = call "Stall Data Flow.vim"("value in"=w47, "milliseconds to wait"=u32 100) -> ("value out"=w46:errorcluster)  [unwired: 1 out]
      n134 = call "CSM Get Module Attribute.vim"("CSM Name"=w6, "Attribute"=w33, "Default Value (Empty Variant)"=0 ("x+1"), "Error In"=w46) -> ("CSM Name (Dup)"=w34:string, "Found"=w44:bool, "Value"=w43:i32, "error out"=w32:errorcluster)  [unwired: 7 in, 1 out]
      n135 = Equal?(x=w39, y=w43) -> (x = y?=w42:bool)
      n136 = And(x=w44, y=w42) -> (x .and. y?=w28:bool)
      n137 = flat-sequence {
        tunnel: w34 -> [w75]
        tunnel: w33 -> [w74]
        tunnel: w32 -> [w73]
        tunnel: [w73] -> w36
        tunnel: [w72] -> w35
        tunnel: w6 -> [w80]
        tunnel: w36 -> [w79]
        tunnel: w35 -> [w78]
        tunnel: [w79] -> w31
        tunnel: [w78] -> w30
        tunnel: [w76] -> w29
        frame #0 {
          n138 = call "CSM - Delete Module Attribute.vi"("CSM Name"=w75, "Attribute"=w74) -> ("error out"=w72:errorcluster)  [unwired: 10 in, 3 out]
        }
        frame #1 {
          n139 = call "CSM - Wait and Send Message for Reply.vi"("State"="Macro: Exit", "Target Module"=w80) -> ("error out"=w77:errorcluster)  [unwired: 10 in, 3 out]
          n140 = call <vilib>:"Clear Errors.vi"("error in (no error)"=w77) -> ("error out"=w76:errorcluster)  [unwired: 5 in, 1 out]
        }
      }
      n141 = Merge Errors(w31, w30, w29) -> (w12:errorcluster)
      n142 = call "Package Error Info.vi"("error in"=w12, "String in"="General Error") -> ("packed error info out"=w13:string, "error status"=w17:bool)  [unwired: 8 in]
      n143 = call-dynamic "failIf.vi"("message (\"\")"=w13, "fail"=w17, "TestCase in"=w16) -> ("error out"=w14:errorcluster, "TestCase out"=w15:refnum<class "testcase-CSMBroadcast.lvclass">)  [unwired: 7 in]
      n144 = call-dynamic "passIf.vi"("error in (no error)"=w14, "message (\"\")"="Before unreigster" ("message (\"\")"), "pass"=w57, "TestCase in"=w15) -> ("error out"=w38:errorcluster, "TestCase out"=w37:refnum<class "testcase-CSMBroadcast.lvclass">)  [unwired: 6 in]
      n145 = call-dynamic "passIf.vi"("error in (no error)"=w38, "message (\"\")"="After unregister" ("message (\"\")"), "pass"=w28, "TestCase in"=w37) -> ("error out"=w20:errorcluster, "TestCase out"=w21:refnum<class "testcase-CSMBroadcast.lvclass">)  [unwired: 6 in]
      n146 = flat-sequence {
        tunnel: w20 -> [w71]
        tunnel: [w70] -> w18
        tunnel: w21 -> [w68]
        tunnel: [w68] -> w19
        frame #0 {
          n147 = call "CSM - Drop Broadcast Registry.vi"() -> ("error out"=w69:errorcluster)  [unwired: 15 in]
          n148 = Merge Errors(w71, w69) -> (w70:errorcluster)
        }
      }
    }
    frame Disabled {
      # "skip test result while test is under development"
      n149 = call <vilib>:"skip.vi"("error in (no error)"=w419, "TestCase in"=w422) -> ("error out"=w421:errorcluster, "TestCase out"=w420:refnum<class "testcase-CSMBroadcast.lvclass">)  [unwired: 8 in]
    }
  }
  "error out" <- w4
  "TestCase out" <- w2
